vi "TLPM Get Average Count.vi"(8 "error in (no error)":errorcluster {"code" format="%.0x"}, 11 "instrument handle":refnum<visa-resource-name>) -> (0 "error out":errorcluster {"code" format="%.0x"}, 2 "Average Count":i16, 3 "instrument handle out":refnum<visa-resource-name>)   [LabVIEW 2019]
doc: "This VI returns the average count for measurement value generation.\n\nNotes:\n(1) The VI is only available on PM100A, PM100D, PM100USB, PM200, PM400.\n(2) The VI is deprecated and kept for legacy reasons. Its recommended to use TLPM Get Average Time.vi() instead."
uses:
  TLPM_32.dll
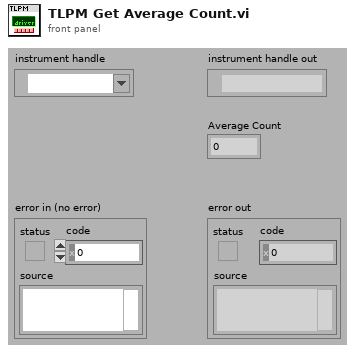
[diagram p1: front panel]
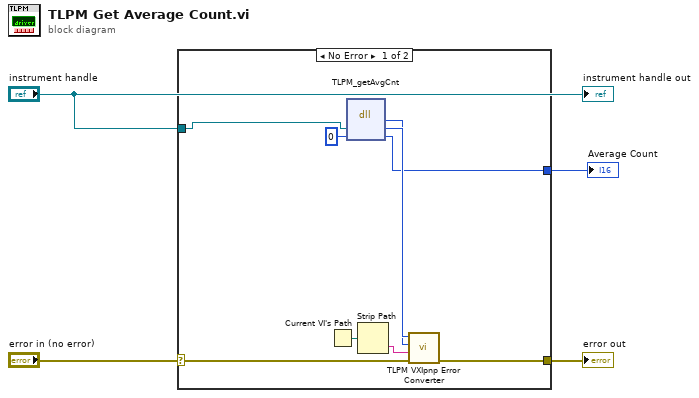
[diagram p0: block diagram]
diagram:
  n1 = case shown="No Error" "error in (no error)" {
    selector: "error in (no error)" -> [w8 w14]
    tunnel: [w7 w14] -> w4
    tunnel: "instrument handle" -> [w12 _]
    tunnel: [w5 _] -> w1
    frame No Error {
      n2 = Current VI's Path() -> (path=w13:path)
      n3 = dll-call lib="TLPM_32.dll" fn="TLPM_getAvgCnt"("Instrument Handle"=w12, "Average Count"=i16 0) -> (w10:i32, "Instrument Handle"=w11:u32, "Average Count"=w5:i16)  [unwired: 3 in, 2 out]
      n4 = Strip Path(path=w13) -> (name=w9:string)  [unwired: 1 out]
      n5 = call <userlib>:"TLPM VXIpnp Error Converter.vi"("error in (no error)"=w8, "Name Of VI (\"\")"=w9, "CVI Error Code (0)"=w10, "instrument handle"=w11) -> ("error out"=w7:errorcluster)  [unwired: 6 in, 1 out]
    }
    frame Error {
    }
  }
  "error out" <- w4
  "Average Count" <- w1
  "instrument handle out" <- "instrument handle"
